vi "Main.vi"(11 "Module Admin":refnum<class "Delacor_lib_QMH_Module Admin.lvclass">) -> ()   [LabVIEW 2016, in "Logger.lvlib"]
doc: "This template is based off of the Queued Message Handler design pattern and the Queued Message Handler project template that ships with LabVIEW.\n\nThe main difference is that the queue is private to this module and communication between modules is performed via Broadcast and Request events.\n\nRequest events are wrapped in public API methods and are handled in the Event Handling Loop (EHL) of this VI. Any module can register for Broadcast events sent by this module. The EHL generates messages based on user interface actions.\n\nThe Message Handling Loop (MHL) processes messages generated by the EHL, or by other messages. The messages are string values, so new messages can be added easily to the Message Cases case structure in the MHL. Each message cluster can also provide an optional value for Message Data, which is a variant that can be converted to whatever message-specific data is required.\n_____\nBased on Delacor QMH Project Template 4.0.0.47.\n_____\nBased on DQMH Project Template 6.1.0.94.\n\n<b>Note:</b> This VI was modified by the <b>Validate DQMH Module</b> tool to add a 'Panel Hidden' status updated broadcast to the Panel Close? event when External Launch = TRUE.\n\n<b>Note:</b> This VI was modified by the <b>Validate DQMH Module</b> tool to add a call to the Error Reported VI at the end of the 'Exit' MHL frame."
uses:
  Logger.lvlib
  <vilib>/Delacor/Delacor QMH/Libraries/Module Admin_class/Delacor_lib_QMH_Module Admin.lvclass
  Module Data--cluster.ctl
  CML Shared/EEG Channel Settings.ctl
  Stop Argument--cluster.ctl
  <vilib>/Delacor/Delacor QMH/Libraries/Message Queue_class/Delacor_lib_QMH_Message Queue.lvclass/Delacor_lib_QMH_Message Queue.ctl
  <vilib>/Delacor/Delacor QMH/Libraries/Module Admin_class/Delacor_lib_QMH_Module Admin.lvclass/Delacor_lib_QMH_Module Admin.ctl
  Initialize File Argument--cluster.ctl
  Initialize File (Reply Payload)--cluster.ctl
  Log Data Argument--cluster.ctl
  Acquisition/WiBCI16T_Data.ctl
  Acquisition/WiBCI16T_Status.ctl
  Acquisition/Reg_Map.ctl
  Stop Logging Argument--cluster.ctl
  Settings Editor/Update Application Settings (Reply Payload)--cluster.ctl
  Settings Editor/Settings--cluster.ctl
  Acquisition/Signal Type--enum.ctl
  Acquisition/Calibration Values--cluster.ctl
  <vilib>/Utility/miscctls.llb/LVPointTypeDef.ctl
  <vilib>/Delacor/Delacor QMH/Libraries/Message Queue_class/Delacor_lib_QMH_Enqueue Message (Single).vi
  <vilib>/Delacor/Delacor QMH/Libraries/Module Admin_class/Delacor_lib_QMH_Get External Launch.vi
  <vilib>/Utility/error.llb/Error Cluster From Error Code.vi
  <vilib>/ErrorRing/Error Ring.xnode
  <vilib>/Delacor/Delacor QMH/Libraries/Message Queue_class/Delacor_lib_QMH_Message Queue.lvclass
  Settings Editor/Settings Editor.lvlib
  Acquisition/Acquisition.lvlib
  CML Shared/CML Shared.lvlib
panel:
  out "Settings":T1={"Log File Base Path"=path "", "Logging"=FALSE, "Text refnum"=refnum, "Log File Full Path"=path "", "EEG Channels"={"16 EEG Channels"=[], "Gain"=24}, "First Log Value"=FALSE} {"EEG Channels"."16 EEG Channels"."Channel No" step=1}
  out "error out":errorcluster
  # "This is a headless module. Show its panel to confirm that the Settings are updated correctly and other debugging tasks. Use the Settings Editor to change the settings for this module."
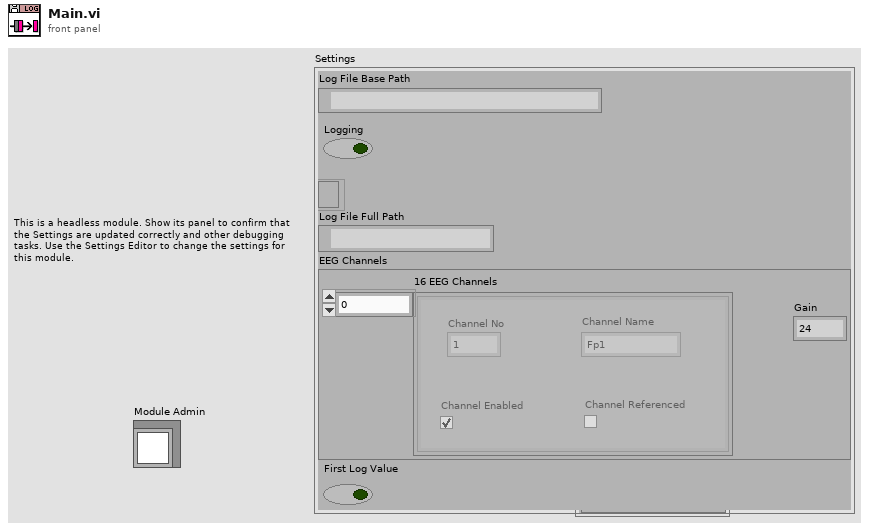
[diagram p1: front panel]
types:
  T1 = typedef "Logger.lvlib/Module Data--cluster.ctl" = cluster{"Log File Base Path":path, "Logging":bool, "Text refnum":refnum<file>, "Log File Full Path":path, "EEG Channels":T2, "First Log Value":bool}
  T2 = typedef "CML Shared.lvlib/EEG Channel Settings.ctl" = cluster{"16 EEG Channels":cluster{"Channel Name":string, "Channel No":u8, "Channel Enabled":bool, "Channel Referenced":bool}[], "Gain":u8}
  T3 = typedef "Settings Editor.lvlib/Broadcast Events--cluster.ctl" = cluster{"Module Did Init":refnum<user-event>, "Status Updated":refnum<user-event>, "Error Reported":refnum<user-event>, "Module Did Stop":refnum<user-event>, "Update Module Execution Status":refnum<user-event>, "Application Settings Updated":refnum<user-event>}
  T4 = typedef "Logger.lvlib/Request Events--cluster.ctl" = cluster{"Stop Module":refnum<user-event>, "Show Panel":refnum<user-event>, "Hide Panel":refnum<user-event>, "Get Module Execution Status":refnum<user-event>, "Show Diagram":refnum<user-event>, "Stop Logging":refnum<user-event>, "Log Data":refnum<user-event>, "Initialize File":refnum<user-event>}
  T5 = enum32{"invalid lock state", "Not Locked", "Locked (No Password)", "Password-protected"}
  T6 = typedef "Logger.lvlib/Stop Argument--cluster.ctl" = cluster{"Origin":string, "Exit via Stop Module Req?":bool, "Wait for Module to stop?":bool}
  T7 = typedef "Logger.lvlib/Initialize File Argument--cluster.ctl" = cluster{"Wait Notifier":refnum<notifier>, "wait for reply":bool, "file name":string}
  T8 = typedef "Logger.lvlib/Log Data Argument--cluster.ctl" = cluster{"WiBCI16T Data out":T9}
  T9 = typedef "Acquisition.lvlib/WiBCI16T_Data.ctl" = cluster{"EEG Ch 1":dbl, "EEG Ch 2":dbl, "EEG Ch 3":dbl, "EEG Ch 4":dbl, "EEG Ch 5":dbl, "EEG Ch 6":dbl, "EEG Ch 7":dbl, "EEG Ch 8":dbl, "EEG Ch 9":dbl, "EEG Ch 10":dbl, "EEG Ch 11":dbl, "EEG Ch 12":dbl, "EEG Ch 13":dbl, "EEG Ch 14":dbl, "EEG Ch 15":dbl, "EEG Ch 16":dbl, "X-Accel":i16, "Y-Accel":i16, "Z-Accel":i16, "X-Gyro":i16, "Y-Gyro":i16, "Z-Gyro":i16, "Timer":u32, "Packet ID":u32, "HW Trig1":u8, "SW Trig1":i8, "HW Trig2":u8, "SW Trig2":i8, "WiBCI Status":T10, "Reg Map":T11}
  T10 = typedef "Acquisition.lvlib/WiBCI16T_Status.ctl" = cluster{"Mode Byte":u8, "Ch Config":u8, "Ch Ref Map":u16, "Ch Enable Map":u16, "Temperature":sgl, "Battery":u8, "Version":string}
  T11 = typedef "Acquisition.lvlib/Reg_Map.ctl" = cluster{"ADS1":u8[], "ADS2":u8[]}
  T12 = typedef "Logger.lvlib/Stop Logging Argument--cluster.ctl" = cluster{"Boolean":bool}
  T13 = typedef "Settings Editor.lvlib/Update Application Settings (Reply Payload)--cluster.ctl" = cluster{"Settings":T14, "error":errorcluster}
  T14 = typedef "Settings Editor.lvlib/Settings--cluster.ctl" = cluster{"Signal Type":T15, "Calibration Array":T16[], "Log File Base Path":path, "EEG Channels":T2, "Soft Trig enum":enum16{"Disable Soft Trigger", "Enable Soft Trigger"}, "Montage selection":cluster{"Montages Ref":refnum<vi>, "Selected Montage Number":u8, "Montages Names":string[]}}
  T15 = typedef "Acquisition.lvlib/Signal Type--enum.ctl" = enum16{"Sine Wave", "Square with Noise"}
  T16 = typedef "Acquisition.lvlib/Calibration Values--cluster.ctl" = cluster{"Slope":dbl, "Offset":dbl}
  T17 = typedef "LVPointTypeDef.ctl" = cluster{"Horizontal":i16, "Vertical":i16}
  T18 = enum32{"Invalid", "Standard", "Closed", "Hidden", "Minimized", "Maximized"}
  T19 = typedef "Logger.lvlib/Initialize File (Reply Payload)--cluster.ctl" = cluster{"File Path":path, "error":errorcluster}
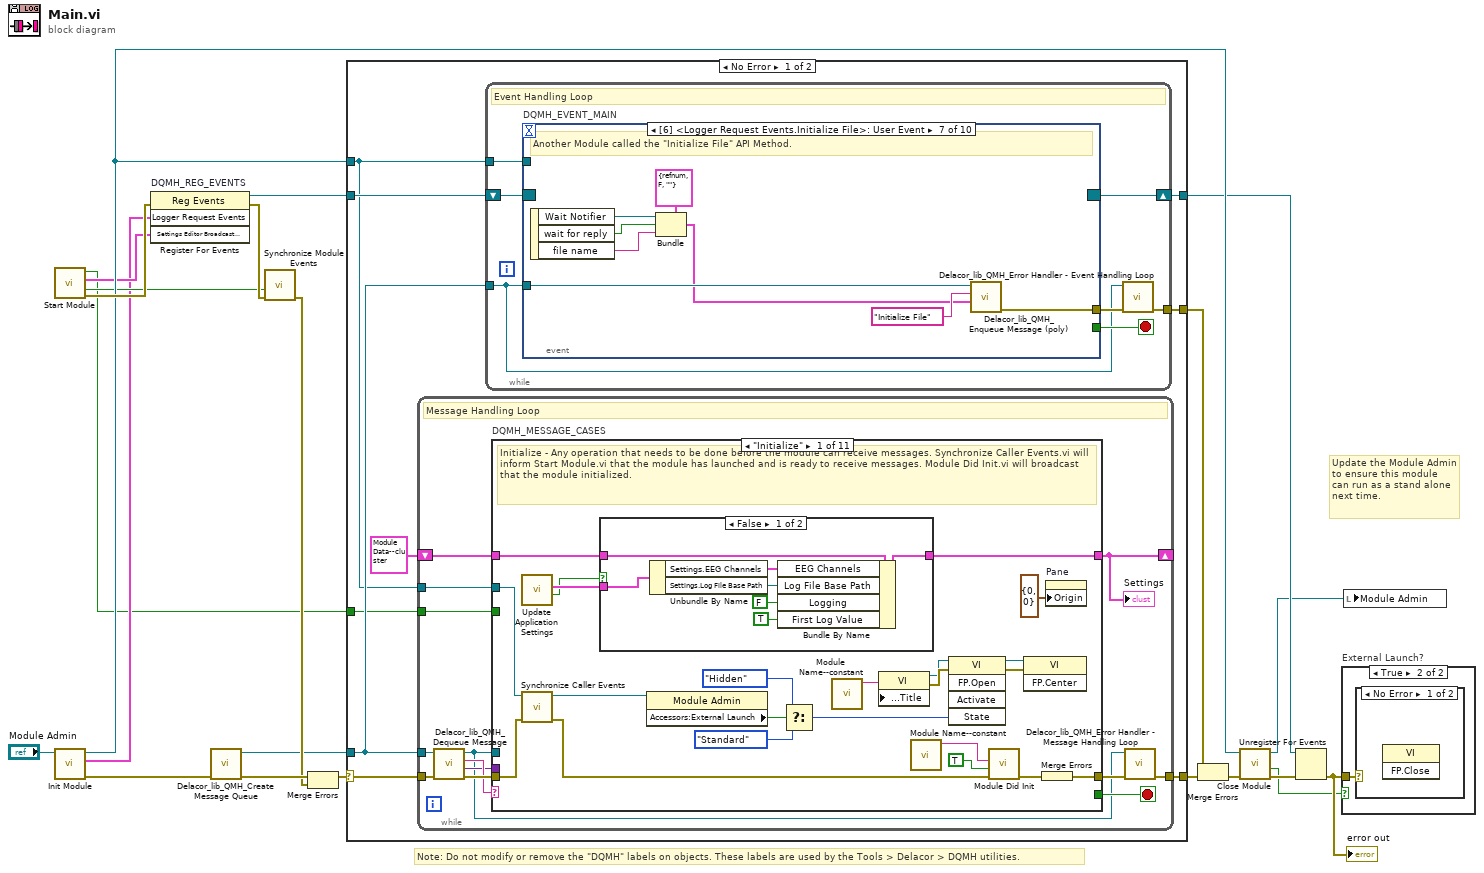
[diagram p0: block diagram]
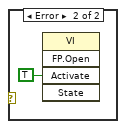
[diagram p3: hidden frame]
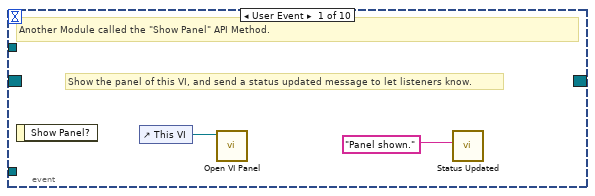
[diagram p4: hidden frame]
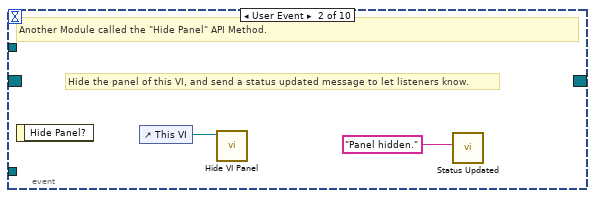
[diagram p5: hidden frame]
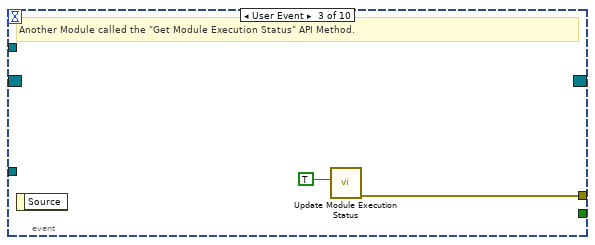
[diagram p6: hidden frame]
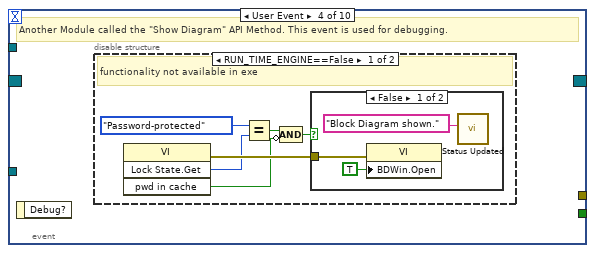
[diagram p7: hidden frame]
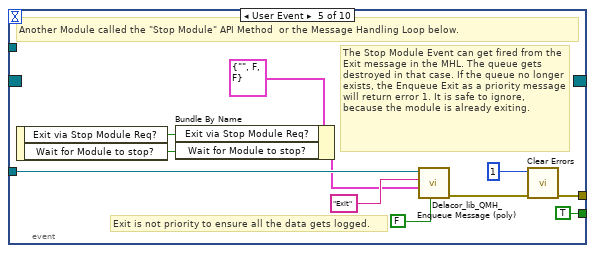
[diagram p10: hidden frame]
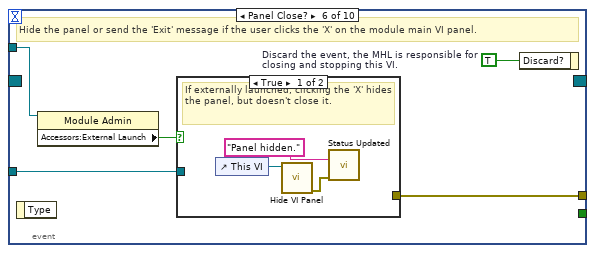
[diagram p11: hidden frame]
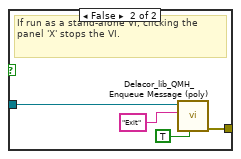
[diagram p12: hidden frame]
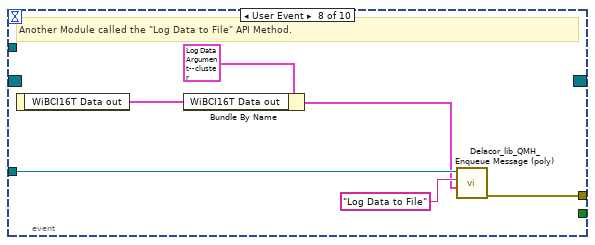
[diagram p13: hidden frame]
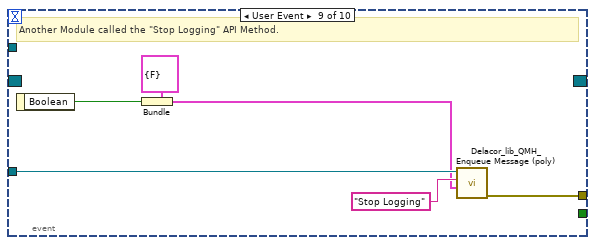
[diagram p14: hidden frame]
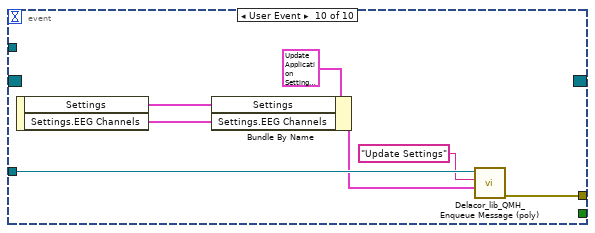
[diagram p15: hidden frame]
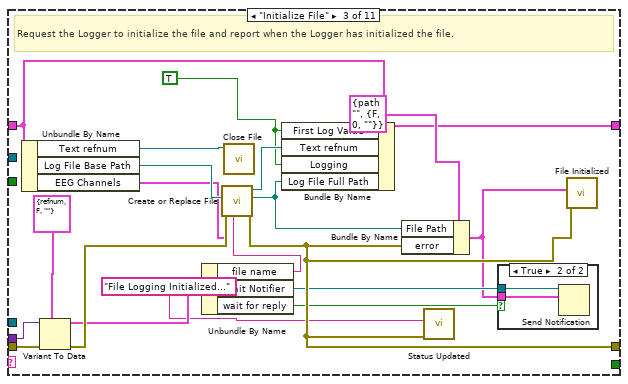
[diagram p18: hidden frame]
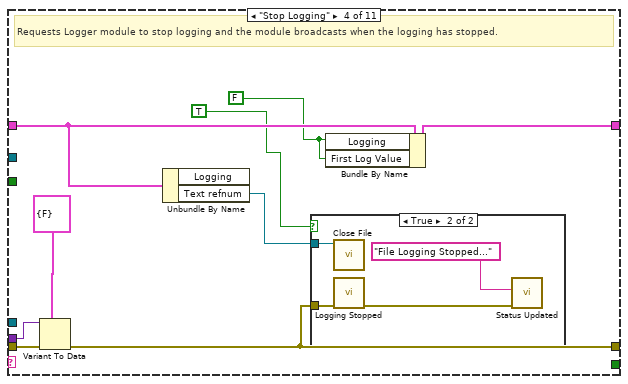
[diagram p20: hidden frame]
diagram:
  # "Note: Do not modify or remove the \"DQMH\" labels on objects. These labels are used by the Tools > Delacor > DQMH utilities."
  # "Update the Module Admin to ensure this module can run as a stand alone next time."
  n1 = call "Start Module.vi"() -> ("error out"=w14:errorcluster, "Wait for Event Sync?"=w4:bool, "Settings Editor Broadcast Events"=w3:T3, "Module Was Already Running?"=w1:bool)  [unwired: 8 in]
  n2 = call "Init Module.vi"("Singleton Module Admin in"="Module Admin") -> ("error out"=w21:errorcluster, "Logger Request Events"=w2:T4, "Singleton Module Admin out"=w11:refnum<class "Delacor_lib_QMH_Module Admin.lvclass">)  [unwired: 8 in]
  n3 = register-events "DQMH_REG_EVENTS"(error in=w14, w2, w3) -> (reference out=w9:refnum<event-registration>, error out=w13:errorcluster)  [unwired: 1 in]
  n4 = call <vilib>:"Delacor_lib_QMH_Create Message Queue.vi"("error in"=w21) -> ("error out"=w16:errorcluster, "Message Queue"=w8:refnum<class "Delacor_lib_QMH_Message Queue.lvclass">)  [unwired: 9 in]
  n5 = call "Synchronize Module Events.vi"("error in (no error)"=w13, "Wait for Event Sync?"=w4) -> ("error out"=w12:errorcluster)  [unwired: 9 in]
  n6 = Merge Errors(w16, w12) -> (w15:errorcluster)
  n7 = case shown="No Error" w15 {
    selector: w15 -> [w29 w270]
    tunnel: [w31 w269] -> w22
    tunnel: [w28 w277] -> w10
    tunnel: w9 -> [w26 w277]
    tunnel: w8 -> [w25 w271]
    tunnel: [w30 _] -> w19
    tunnel: w11 -> [w24 w273]
    tunnel: w1 -> [w23 w272]
    frame No Error {
      n8 = while {
        tunnel: w25 -> [w107]
        shift-right: [w111] -> _
        shift-left: T1 {"Log File Base Path"=path "", "Logging"=FALSE, "Text refnum"=refnum, "Log File Full Path"=path "", "EEG Channels"={"16 EEG Channels"=[], "Gain"=24}, "First Log Value"=FALSE} ("Data Cluster") -> [w112]
        tunnel: w29 -> [w115]
        tunnel: [w113] -> w31
        tunnel: w24 -> [w105]
        tunnel: w23 -> [w104]
        stop <- w110 stop-if-true
        # "Message Handling Loop"
        n9 = call-dynamic "Delacor_lib_QMH_Dequeue Message.vi"("error in"=w115, "Message Queue in"=w107) -> ("error out"=w114:errorcluster, "Message Data"=w108:variant, "Message"=w109:string, "Message Queue out"=w106:refnum<class "Delacor_lib_QMH_Message Queue.lvclass">)  [unwired: 6 in]
        n10 = case "DQMH_MESSAGE_CASES" shown="\"Initialize\"" w109 {
          selector: w109 -> [_ _ _ _ _ _ _ _ _ _ w256]
          tunnel: w106 -> [_ _ _ _ _ _ _ _ w222 w246 _]
          tunnel: w114 -> [w136 w148 w167 w179 w193 w207 w217 w219 w229 w252 w258]
          tunnel: [w133 w148 w168 w178 w186 w205 w216 w219 w225 w249 w259] -> w116
          tunnel: w112 -> [w124 w147 w157 w175 w192 w197 w215 w218 w224 w238 w257]
          tunnel: [w118 w147 w156 w173 w190 w196 w215 w218 w224 w238 w257] -> w111
          tunnel: [_ _ _ _ _ _ _ _ _ w245 _] -> w110
          tunnel: w108 -> [_ _ w165 w177 w191 w204 _ _ w223 w244 _]
          tunnel: w105 -> [w125 _ _ _ _ _ _ _ w221 w239 _]
          tunnel: w104 -> [_ _ _ _ _ _ _ _ _ w237 _]
          frame "Initialize" {
            # "Initialize - Any operation that needs to be done before the module can receive messages. Synchronize Caller Events.vi will inform Start Module.vi that the module has launched and is ready to receive messages. Module Did Init.vi will broadcast that the module initialized."
            n11 = call "Update Application Settings.vi"() -> ("timed out?"=w117:bool, "Reply Payload"=w119:T13)  [unwired: 9 in, 1 out]
            n12 = call "Synchronize Caller Events.vi"("error in (no error)"=w136, "Singleton Module Admin in"=w125) -> ("error out"=w135:errorcluster, "Singleton Module Admin out"=w121:refnum<class "Delacor_lib_QMH_Module Admin.lvclass">)  [unwired: 8 in]
            n13 = case shown="False" w117 {
              tunnel: w124 -> [w145 w146]
              tunnel: w119 -> [w144 _]
              tunnel: [w143 w146] -> w118
              frame False {
                n14 = Unbundle By Name(w144) -> ("Settings.EEG Channels"=w140:T2, "Settings.Log File Base Path"=w142:path)
                n15 = Bundle By Name(cluster=w145, "EEG Channels"=w140, "Log File Base Path"=w142, "Logging"=FALSE, "First Log Value"=TRUE) -> (w143:T1)
              }
              frame True {
              }
            }
            n16 = property class="Module Admin"(reference=w121) -> ("Accessors:External Launch"=w129:bool)  [unwired: 1 in, 2 out]
            n17 = Select(t=T18."Hidden" ("State"), s=w129, f=T18."Standard" ("State")) -> (s? t:f=w126:T18)
            n18 = call "Module Name--constant.vi"() -> ("Module Name"=w132:string)  [unwired: 11 in]
            n19 = property class="VI"("Front Panel.Title"=w132) -> (reference out=w131:refnum<vi>, error out=w138:errorcluster)  [unwired: 2 in]
            n20 = call "Module Name--constant.vi"() -> ("Module Name"=w122:string)  [unwired: 11 in]
            n21 = invoke class="VI" method="FP.Open"(reference=w131, error in=w138, "State"=w126) -> (reference out=w130:refnum<vi>, error out=w137:errorcluster)  [unwired: 2 in, 3 out]
            n22 = call "Module Did Init.vi"("error in (no error)"=w135, "Initialized?"=TRUE, "Origin"=w122) -> ("error out"=w134:errorcluster)  [unwired: 8 in]
            n23 = invoke class="VI" method="FP.Center"(reference=w130, error in=w137) -> ()  [unwired: 1 in, 3 out]
            n24 = Merge Errors(w134) -> (w133:errorcluster)
            n25 = property on="Pane" class="Pane"("Origin"=T17 {"Horizontal"=0, "Vertical"=0}) -> ()  [unwired: 2 in, 2 out]
          }
          frame "---Module Specific---" {
            # "Separator -- The following cases handle messages specific to this Module."
          }
          frame "Initialize File" {
            w150 = TRUE ("Logging")
            # "Request the Logger to initialize the file and report when the Logger has initialized the file."
            n26 = Unbundle By Name(w157) -> ("Text refnum"=w154:refnum<file>, "Log File Base Path"=w158:path, "EEG Channels"=w151:T2)
            n27 = Variant To Data(error in=w167, type=T7 {"Wait Notifier"=refnum, "wait for reply"=FALSE, "file name"=""} ("Initialize File Argument"), Variant=w165) -> (data=w163:T7, error out=w166:errorcluster)
            n28 = Unbundle By Name(w163) -> ("file name"=w149:string, "Wait Notifier"=w162:refnum<notifier>, "wait for reply"=w161:bool)
            n29 = call "Create or Replace File.vi"("file name"=w149, "error in"=w166, "EEG Channels"=w151, "Log File Base Path"=w158) -> ("error out"=w168:errorcluster, "File Path"=w152:path, "Text refnum"=w153:refnum<file>)  [unwired: 5 in]
            n30 = call "Close File.vi"("Text refnum"=w154) -> ()  [unwired: 10 in, 1 out]
            n31 = Bundle By Name(cluster=w157, "First Log Value"=w150, "Text refnum"=w153, "Logging"=w150, "Log File Full Path"=w152) -> (w156:T1)
            n32 = Bundle By Name(cluster=T19 {"File Path"=path "", "error"={"status"=FALSE, "code"=0, "source"=""}} ("Initialize File (Reply Payload)"), "File Path"=w152, "error"=w168) -> (w159:T19)
            n33 = call "Status Updated.vi"("error in (no error)"=w168, "Status"="File Logging Initialized...") -> ()  [unwired: 9 in, 1 out]
            n34 = case shown="True" w161 {
              tunnel: w162 -> [_ w170]
              tunnel: w159 -> [_ w169]
              frame False {
              }
              frame True {
                n35 = Send Notification(notification=w169, notifier=w170) -> ()  [unwired: 1 in, 2 out]
              }
            }
            n36 = call "File Initialized.vi"("error in (no error)"=w168, "Reply Payload"=w159) -> ()  [unwired: 9 in, 1 out]
          }
          frame "Stop Logging" {
            w171 = FALSE ("Logging")
            # "Requests Logger module to stop logging and the module broadcasts when the logging has stopped."
            n37 = Variant To Data(error in=w179, type=T12 {"Boolean"=FALSE} ("Stop Logging Argument"), Variant=w177) -> (error out=w178:errorcluster)  [unwired: 1 out]
            n38 = Unbundle By Name(w175) -> ("Text refnum"=w174:refnum<file>)  [unwired: 1 out]
            n39 = case shown="True" TRUE {
              tunnel: w178 -> [_ w183]
              tunnel: w174 -> [_ w180]
              frame False {
                # "We were not logging, so this is a no-op."
              }
              frame True {
                n40 = call "Close File.vi"("Text refnum"=w180) -> ()  [unwired: 10 in, 1 out]
                n41 = call "Logging Stopped.vi"("error in (no error)"=w183) -> ("error out"=w182:errorcluster)  [unwired: 10 in]
                n42 = call "Status Updated.vi"("error in (no error)"=w182, "Status"="File Logging Stopped...") -> ()  [unwired: 9 in, 1 out]
              }
            }
            n43 = Bundle By Name(cluster=w175, "Logging"=w171, "First Log Value"=w171) -> (w173:T1)
          }
          frame "Update Settings" {
            n44 = Variant To Data(error in=w193, type=T13 {"Settings"={"Signal Type"=enum."Sine Wave", "Calibration Array"=[], "Log File Base Path"=path "", "EEG Channels"={"16 EEG Channels"=[], "Gain"=24}, "Soft Trig enum"=enum."Disable Soft Trigger", "Montage selection"={"Montages Ref"=refnum, "Selected Montage Number"=0, "Montages Names"=[]}}, "error"={"status"=FALSE, "code"=0, "source"=""}} ("Settings Updated Argument"), Variant=w191) -> (data=w189:T13, error out=w186:errorcluster)
            n45 = Unbundle By Name(w189) -> ("Settings.EEG Channels"=w184:T2, "Settings.Log File Base Path"=w188:path)
            n46 = Bundle By Name(cluster=w192, "EEG Channels"=w184, "Log File Base Path"=w188) -> (w190:T1)
            n47 = call "Status Updated.vi"("error in (no error)"=w186, "Status"="Settings Updated") -> ()  [unwired: 9 in, 1 out]
          }
          frame "Log Data to File" {
            # "Requests Logger module to log data to file"
            n48 = Variant To Data(error in=w207, type=T8 {"WiBCI16T Data out"={"EEG Ch 1"=0.0, "EEG Ch 2"=0.0, "EEG Ch 3"=0.0, "EEG Ch 4"=0.0, "EEG Ch 5"=0.0, "EEG Ch 6"=0.0, "EEG Ch 7"=0.0, "EEG Ch 8"=0.0, "EEG Ch 9"=0.0, "EEG Ch 10"=0.0, "EEG Ch 11"=0.0, "EEG Ch 12"=0.0, "EEG Ch 13"=0.0, "EEG Ch 14"=0.0, "EEG Ch 15"=0.0, "EEG Ch 16"=0.0, "X-Accel"=0, "Y-Accel"=0, "Z-Accel"=0, "X-Gyro"=0, "Y-Gyro"=0, "Z-Gyro"=0, "Timer"=0, "Packet ID"=0, "HW Trig1"=0, "SW Trig1"=0, "HW Trig2"=0, "SW Trig2"=0, "WiBCI Status"={"Mode Byte"=0, "Ch Config"=0, "Ch Ref Map"=0, "Ch Enable Map"=0, "Temperature"=0.0, "Battery"=0, "Version"=""}, "Reg Map"={"ADS1"=[], "ADS2"=[]}}} ("Log Data to File Argument"), Variant=w204) -> (data=w202:T8, error out=w206:errorcluster)
            n49 = Unbundle By Name(w197) -> ("First Log Value"=w194:bool, "Logging"=w199:bool, "Text refnum"=w200:refnum<file>, "Log File Full Path"=w198:path)
            n50 = Unbundle By Name(w202) -> ("WiBCI16T Data out"=w201:T9)
            n51 = Bundle By Name(cluster=w197, "First Log Value"=FALSE) -> (w196:T1)
            n52 = case shown="True" w199 {
              tunnel: w206 -> [w208 w214]
              tunnel: [w208 w213] -> w205
              tunnel: w201 -> [_ w210]
              tunnel: w200 -> [_ w211]
              tunnel: w198 -> [_ w212]
              tunnel: w194 -> [_ w209]
              frame False {
                # "We are not currently logging, so this action is a no-op."
              }
              frame True {
                n53 = call "Log Data to File.vi"("First Log Value"=w209, "error in"=w214, "WiBCI16T Data out"=w210, "file path"=w212, "Text refnum"=w211) -> ("error out"=w213:errorcluster)  [unwired: 6 in]
              }
            }
          }
          frame "---Copy This Frame---" {
            # "Duplicate this frame when creating new messages.  Change this comment in the duplicated frame to describe this message."
            n54 = Merge Errors(w217) -> (w216:errorcluster)
          }
          frame "---Exit and Error Handling---" {
            # "Separator - The following cases handle errors and exit messages."
          }
          frame "Error" {
            # "Error - Check the error message data and respond accordingly. This message is sent by the \"Error Handler\" VIs at the end of each loop in this application."
            n55 = Variant To Data(error in=w229, type=errorcluster {"status"=FALSE, "code"=0, "source"=""} ("error constant"), Variant=w223) -> (data=w230:errorcluster, error out=w227:errorcluster)
            n56 = property class="Module Admin"(reference=w221) -> ("Accessors:External Launch"=w220:bool)  [unwired: 1 in, 2 out]
            n57 = call "Error Reported.vi"("Error"=w230) -> ()  [unwired: 10 in, 1 out]
            n58 = case shown="False" w220 {
              tunnel: [w235 _] -> w226
              tunnel: w222 -> [w233 _]
              tunnel: w230 -> [w234 _]
              frame False {
                # "If the module is running standalone, then pop up an error dialog and call the \"Exit\" message."
                n59 = call <vilib>:"Simple Error Handler.vi"("error in (no error)"=w234) -> ()  [unwired: 4 in, 5 out]
                n60 = call-poly <vilib>:"Delacor_lib_QMH_Enqueue Message (poly).vi"("Priority Message? (F)"=TRUE, "Message"="Exit", "Message Queue in"=w233) -> ("error out"=w235:errorcluster)  [unwired: 7 in, 1 out]
              }
              frame True {
                # "If the module was launched externally, calling the Error Reported broadcast VI is the only action performed by the \"Error\" message. The module's caller can then process the error appropriately."
              }
            }
            n61 = Merge Errors(w227, w226) -> (w225:errorcluster)
            n62 = local write "error out"(w225) -> ()
          }
          frame "Exit" {
            w243 = 91  # 91: not all Exit messages will have an argument
            w245 = TRUE  # Stop the VI
            # "Release the message queue reference"
            # "Exit - Exit the application."
            n63 = Variant To Data(error in=w252, type=T6 {"Origin"="", "Exit via Stop Module Req?"=FALSE, "Wait for Module to stop?"=FALSE} ("Stop Argument"), Variant=w244) -> (data=w241:T6, error out=w248:errorcluster)
            n64 = call <vilib>:"Clear Errors.vi"("error in (no error)"=w248, "specific error code to clear (0: all)"=w243) -> ("error out"=w251:errorcluster)  [unwired: 4 in, 1 out]
            n65 = Unbundle By Name(w238) -> ("Text refnum"=w236:refnum<file>)
            n66 = control-ref of="This VI"() -> (w240:refnum<vi>)
            n67 = call-dynamic "Delacor_lib_QMH_Release Message Queue.vi"("error in"=w251, "Message Queue"=w246) -> ("error out"=w250:errorcluster)  [unwired: 9 in]
            n68 = call "Handle Exit.vi"("Stop Argument"=w241, "Admin in"=w239, "VI reference"=w240) -> ("error out"=w247:errorcluster)  [unwired: 7 in, 1 out]
            n69 = call "Close File.vi"("Text refnum"=w236) -> ()  [unwired: 10 in, 1 out]
            n70 = case "Settings Editor was\nalready running?" shown="False" w237 {
              frame False {
                n71 = call "Module Name--constant.vi"() -> ("Module Name"=w254:string)  [unwired: 11 in]
                n72 = call "Stop Module.vi"("Wait for Module to Stop? (F)"=TRUE, "Origin"=w254) -> ()  [unwired: 9 in, 1 out]
              }
              frame True {
                # "Another Module is\nin charge of stopping Settings Editor"
              }
            }
            n73 = Merge Errors(w250, w247) -> (w249:errorcluster)
            n74 = call "Error Reported.vi"("Error"=w249) -> ()  [unwired: 10 in, 1 out]
          }
          frame Default {
            # "'Default' case only runs if there is a message that isn't defined in any of the other cases.  Output a programming error."
            n75 = call "Module Name--constant.vi"() -> ("Module Name"=w255:string)  [unwired: 11 in]
            n76 = xnode "Error Ring"("parameter 0"=w256, "parameter 1"=w255) -> ("error out"=w260:errorcluster)
            n77 = Merge Errors(w258, w260) -> (w259:errorcluster)
          }
        }
        "Settings" <- w111
        n78 = call-dynamic "Delacor_lib_QMH_Error Handler - Message Handling Loop.vi"("error in"=w116, "Message Queue in"=w106) -> ("dup error in"=w113:errorcluster)  [unwired: 8 in, 1 out]
      }
      n79 = while {
        tunnel: w25 -> [w32]
        shift-right: [w35] -> w28
        shift-left: w26 -> [w36]
        tunnel: [w37] -> w30
        tunnel: w24 -> [w33]
        stop <- w34 stop-if-true
        # "Event Handling Loop"
        n80 = event "DQMH_EVENT_MAIN" shown="[6] <Logger Request Events.Initialize File>: User Event" {
          selector: w36 -> [_ _ _ _ _ _ _ _ _ _]
          dyn-events: [_ _ _ _ _ _ _ _ _ _] -> w35
          timeout: _ -> [_ _ _ _ _ _ _ _ _ _]
          tunnel: [_ _ _ _ TRUE ("Discard?") _ _ _ _ _] -> w34
          tunnel: w32 -> [_ _ _ _ w60 w67 w83 w89 w95 w102]
          tunnel: [_ _ w44 _ w63 w69 w84 w90 w96 w103] -> w38
          tunnel: w33 -> [_ _ _ _ _ w66 _ _ _ _]
          event User Event {
            # "Show the panel of this VI, and send a status updated message to let listeners know."
            # "Another Module called the \"Show Panel\" API Method."
            n81 = event-data() -> ()  [unwired: 1 in, 1 out]
            n82 = control-ref of="This VI"() -> (w40:refnum<vi>)
            n83 = call "Open VI Panel.vi"("VI"=w40) -> ()  [unwired: 10 in, 1 out]
            n84 = call "Status Updated.vi"("Status"="Panel shown." ("format string")) -> ()  [unwired: 10 in, 1 out]
          }
          event User Event {
            # "Hide the panel of this VI, and send a status updated message to let listeners know."
            # "Another Module called the \"Hide Panel\" API Method."
            n85 = event-data() -> ()  [unwired: 1 in, 1 out]
            n86 = control-ref of="This VI"() -> (w42:refnum<vi>)
            n87 = call "Hide VI Panel.vi"("VI"=w42) -> ()  [unwired: 10 in, 1 out]
            n88 = call "Status Updated.vi"("Status"="Panel hidden." ("format string")) -> ()  [unwired: 10 in, 1 out]
          }
          event User Event {
            # "Another Module called the \"Get Module Execution Status\" API Method."
            n89 = event-data() -> ()  [unwired: 1 in, 1 out]
            n90 = call "Update Module Execution Status.vi"("Running?"=TRUE) -> ("error out"=w44:errorcluster)  [unwired: 10 in]
          }
          event User Event {
            # "Another Module called the \"Show Diagram\" API Method. This event is used for debugging."
            n91 = event-data() -> ()  [unwired: 1 in, 1 out]
            n92 = disable-structure shown="RUN_TIME_ENGINE==False" {
              frame condition #0 (active) {
                # "functionality not available in exe"
                n93 = invoke class="VI" method="Lock State.Get"() -> (error out=w50:errorcluster, "Get Lock State"=w49:T5, "pwd in cache"=w46:bool)  [unwired: 4 in, 1 out]
                n94 = Equal?(x=T5."Password-protected", y=w49) -> (x = y?=w47:bool)
                n95 = Compound Arithmetic op=AND(w47, invert w46) -> (w45:bool)
                n96 = case shown="False" w45 {
                  tunnel: w50 -> [w53 _]
                  frame False {
                    n97 = property class="VI"(error in=w53, "BDWin.Open"=TRUE ("Block Diagram Window:Open")) -> ()  [unwired: 1 in, 2 out]
                    n98 = call "Status Updated.vi"("Status"="Block Diagram shown." ("format string")) -> ()  [unwired: 10 in, 1 out]
                  }
                  frame True {
                    # "Password-protected VI, and the password is not in the cache. Do not show the diagram."
                  }
                }
              }
              frame condition #1 {
              }
            }
          }
          event User Event {
            # "Exit is not priority to ensure all the data gets logged."
            # "The Stop Module Event can get fired from the Exit message in the MHL. The queue gets destroyed in that case. If the queue no longer exists, the Enqueue Exit as a priority message will return error 1. It is safe to ignore, because the module is already exiting."
            # "Another Module called the \"Stop Module\" API Method  or the Message Handling Loop below."
            n99 = event-data() -> ("Exit via Stop Module Req?"=w56:bool, "Wait for Module to stop?"=w55:bool)  [unwired: 1 in]
            n100 = Bundle By Name(cluster=T6 {"Origin"="", "Exit via Stop Module Req?"=FALSE, "Wait for Module to stop?"=FALSE} ("Stop Argument"), "Exit via Stop Module Req?"=w56, "Wait for Module to stop?"=w55) -> (w54:T6)
            n101 = call-poly <vilib>:"Delacor_lib_QMH_Enqueue Message (poly).vi"("Priority Message? (F)"=FALSE, "Message Data"=w54, "Message"="Exit", "Message Queue in"=w60) -> ("error out"=w64:errorcluster)  [unwired: 6 in, 1 out]
            n102 = call <vilib>:"Clear Errors.vi"("error in (no error)"=w64, "specific error code to clear (0: all)"=1) -> ("error out"=w63:errorcluster)  [unwired: 4 in, 1 out]
          }
          event Panel Close? {
            w68 = TRUE  # Discard the event, the MHL is responsible for closing and stopping this VI.
            # "Hide the panel or send the 'Exit' message if the user clicks the 'X' on the module main VI panel."
            n103 = event-data() -> ()  [unwired: 1 in, 1 out]
            n104 = property class="Module Admin"(reference=w66) -> ("Accessors:External Launch"=w65:bool)  [unwired: 1 in, 2 out]
            n105 = case shown="True" w65 {
              tunnel: w67 -> [_ w75]
              tunnel: [_ w76] -> w69
              frame True {
                # "If externally launched, clicking the 'X' hides the panel, but doesn't close it."
                n106 = control-ref of="This VI"() -> (w72:refnum<vi>)
                n107 = call "Hide VI Panel.vi"("VI"=w72) -> ("error out"=w70:errorcluster)  [unwired: 10 in]
                n108 = call "Status Updated.vi"("error in (no error)"=w70, "Status"="Panel hidden.") -> ()  [unwired: 9 in, 1 out]
              }
              frame False {
                # "If run as a stand-alone VI, clicking the panel 'X' stops the VI."
                n109 = call-poly <vilib>:"Delacor_lib_QMH_Enqueue Message (poly).vi"("Priority Message? (F)"=TRUE, "Message"="Exit", "Message Queue in"=w75) -> ("error out"=w76:errorcluster)  [unwired: 7 in, 1 out]
              }
            }
            n110 = event-data("Discard?"=w68) -> ()  [unwired: 1 in, 1 out]
          }
          event User Event {
            # "Another Module called the \"Initialize File\" API Method."
            n111 = event-data() -> ("Wait Notifier"=w79:refnum<notifier>, "wait for reply"=w78:bool, "file name"=w77:string)  [unwired: 1 in]
            n112 = Bundle(cluster=T7 {"Wait Notifier"=refnum, "wait for reply"=FALSE, "file name"=""} ("Initialize File Argument"), "Wait Notifier"=w79, "wait for reply"=w78, "file name"=w77) -> (w80:T7)
            n113 = call-poly <vilib>:"Delacor_lib_QMH_Enqueue Message (poly).vi"("Message Data"=w80, "Message"="Initialize File", "Message Queue in"=w83) -> ("error out"=w84:errorcluster)  [unwired: 7 in, 1 out]
          }
          event User Event {
            # "Another Module called the \"Log Data to File\" API Method."
            n114 = event-data() -> ("WiBCI16T Data out"=w86:T9)  [unwired: 1 in]
            n115 = Bundle By Name(cluster=T8 {"WiBCI16T Data out"={"EEG Ch 1"=0.0, "EEG Ch 2"=0.0, "EEG Ch 3"=0.0, "EEG Ch 4"=0.0, "EEG Ch 5"=0.0, "EEG Ch 6"=0.0, "EEG Ch 7"=0.0, "EEG Ch 8"=0.0, "EEG Ch 9"=0.0, "EEG Ch 10"=0.0, "EEG Ch 11"=0.0, "EEG Ch 12"=0.0, "EEG Ch 13"=0.0, "EEG Ch 14"=0.0, "EEG Ch 15"=0.0, "EEG Ch 16"=0.0, "X-Accel"=0, "Y-Accel"=0, "Z-Accel"=0, "X-Gyro"=0, "Y-Gyro"=0, "Z-Gyro"=0, "Timer"=0, "Packet ID"=0, "HW Trig1"=0, "SW Trig1"=0, "HW Trig2"=0, "SW Trig2"=0, "WiBCI Status"={"Mode Byte"=0, "Ch Config"=0, "Ch Ref Map"=0, "Ch Enable Map"=0, "Temperature"=0.0, "Battery"=0, "Version"=""}, "Reg Map"={"ADS1"=[], "ADS2"=[]}}} ("Log Data to File Argument"), "WiBCI16T Data out"=w86) -> (w85:T8)
            n116 = call-poly <vilib>:"Delacor_lib_QMH_Enqueue Message (poly).vi"("Message Data"=w85, "Message"="Log Data to File", "Message Queue in"=w89) -> ("error out"=w90:errorcluster)  [unwired: 7 in, 1 out]
          }
          event User Event {
            # "Another Module called the \"Stop Logging\" API Method."
            n117 = event-data() -> ("Boolean"=w91:bool)  [unwired: 1 in]
            n118 = Bundle(cluster=T12 {"Boolean"=FALSE} ("Stop Logging Argument"), "Boolean"=w91) -> (w92:T12)
            n119 = call-poly <vilib>:"Delacor_lib_QMH_Enqueue Message (poly).vi"("Message Data"=w92, "Message"="Stop Logging", "Message Queue in"=w95) -> ("error out"=w96:errorcluster)  [unwired: 7 in, 1 out]
          }
          event User Event {
            n120 = event-data() -> ("Settings"=w99:T14, "Settings.EEG Channels"=w97:T2)  [unwired: 1 in]
            n121 = Bundle By Name(cluster=T13 {"Settings"={"Signal Type"=enum."Sine Wave", "Calibration Array"=[], "Log File Base Path"=path "", "EEG Channels"={"16 EEG Channels"=[], "Gain"=24}, "Soft Trig enum"=enum."Disable Soft Trigger", "Montage selection"={"Montages Ref"=refnum, "Selected Montage Number"=0, "Montages Names"=[]}}, "error"={"status"=FALSE, "code"=0, "source"=""}} ("Settings Updated Argument"), "Settings"=w99, "Settings.EEG Channels"=w97) -> (w98:T13)
            n122 = call-poly <vilib>:"Delacor_lib_QMH_Enqueue Message (poly).vi"("Message Data"=w98, "Message"="Update Settings", "Message Queue in"=w102) -> ("error out"=w103:errorcluster)  [unwired: 7 in, 1 out]
          }
        }
        n123 = call-dynamic "Delacor_lib_QMH_Error Handler - Event Handling Loop.vi"("error in"=w38, "Message Queue in"=w32) -> ("dup error in"=w37:errorcluster)  [unwired: 8 in, 1 out]
      }
    }
    frame Error {
      # "Synchronize Caller Events.vi will inform Start Module.vi that the module has launched and will let the code calling Start Module.vi register for broadcasts and would permit the caller receive the broadcast that an error occurred at launch time."
      n124 = call "Synchronize Caller Events.vi"("Singleton Module Admin in"=w273) -> ("error out"=w278:errorcluster)  [unwired: 9 in, 1 out]
      n125 = call-dynamic "Delacor_lib_QMH_Release Message Queue.vi"("error in"=w270, "Message Queue"=w271) -> ("error out"=w269:errorcluster)  [unwired: 9 in]
      n126 = call "Module Name--constant.vi"() -> ("Module Name"=w276:string)  [unwired: 11 in]
      n127 = case "Settings Editor was\nalready running?" shown="False" w272 {
        frame False {
          n128 = call "Module Name--constant.vi"() -> ("Module Name"=w281:string)  [unwired: 11 in]
          n129 = call "Stop Module.vi"("Wait for Module to Stop? (F)"=TRUE, "Origin"=w281) -> ()  [unwired: 9 in, 1 out]
        }
        frame True {
          # "Another Module is\nin charge of stopping Settings Editor"
        }
      }
      n130 = Format Into String(format string="An error occurred during initialization. %s is no longer running.", w276) -> (resulting string=w274:string)  [unwired: 2 in, 1 out]
      n131 = Merge Errors(w270, w278) -> (w279:errorcluster)
      n132 = call "Error Reported.vi"("Additional Information"=w274, "Error"=w279) -> ()  [unwired: 9 in, 1 out]
    }
  }
  n133 = Merge Errors(w19, w22) -> (w18:errorcluster)
  n134 = call "Close Module.vi"("error in (no error)"=w18, "Module Admin in"=w11) -> ("error out"=w20:errorcluster, "External Launch"=w5:bool, "Module Admin out"=w6:refnum<class "Delacor_lib_QMH_Module Admin.lvclass">)  [unwired: 7 in]
  n135 = Unregister For Events(event registration refnum=w10, error in=w20) -> (error out=w17:errorcluster)
  "error out" <- w17
  n136 = case "External Launch?" shown="True" w5 {
    tunnel: w17 -> [_ w282]
    frame False {
    }
    frame True {
      n137 = case shown="No Error" w282 {
        frame No Error {
          n138 = invoke class="VI" method="FP.Close"() -> ()  [unwired: 3 in, 3 out]
        }
        frame Error {
          n139 = invoke class="VI" method="FP.Open"("Activate"=TRUE ("Activate?")) -> ()  [unwired: 4 in, 5 out]
        }
      }
    }
  }
  n140 = local write "Module Admin"(w6) -> ()
